vi "Add Item to Tree.vi"(7 "Tree ref":refnum<vi>, 8 "error in (no error)":errorcluster, 9 "TreeItems (to add)":T1[](array[typedef]), 10 "Insertion index":i32, 11 "TreeItems (current)":T1[](array[typedef])) -> (0 "error out":errorcluster, 3 "TreeItems (added)":T1[](array[typedef]))   [LabVIEW 2020, in "BetterDragAndDrop.lvlib" / "BetterTreeHandle.lvclass"]
uses:
  BetterTreeHandle/BetterTreeHandle.lvclass
  TreeItem.ctl
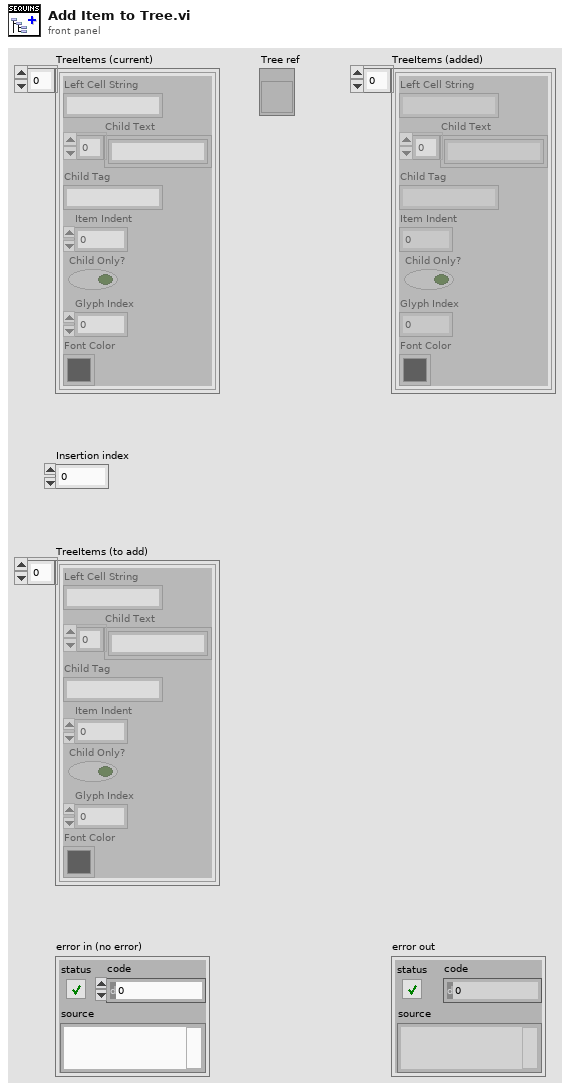
[diagram p1: front panel]
types:
  T1 = typedef "BetterDragAndDrop.lvlib/BetterTreeHandle.lvclass/TreeItem.ctl" = cluster{"Left Cell String":string, "Child Text":string[], "Child Tag":string, "Item Indent":i32, "Child Only?":bool, "Glyph Index":i32, "Font Color":u32}
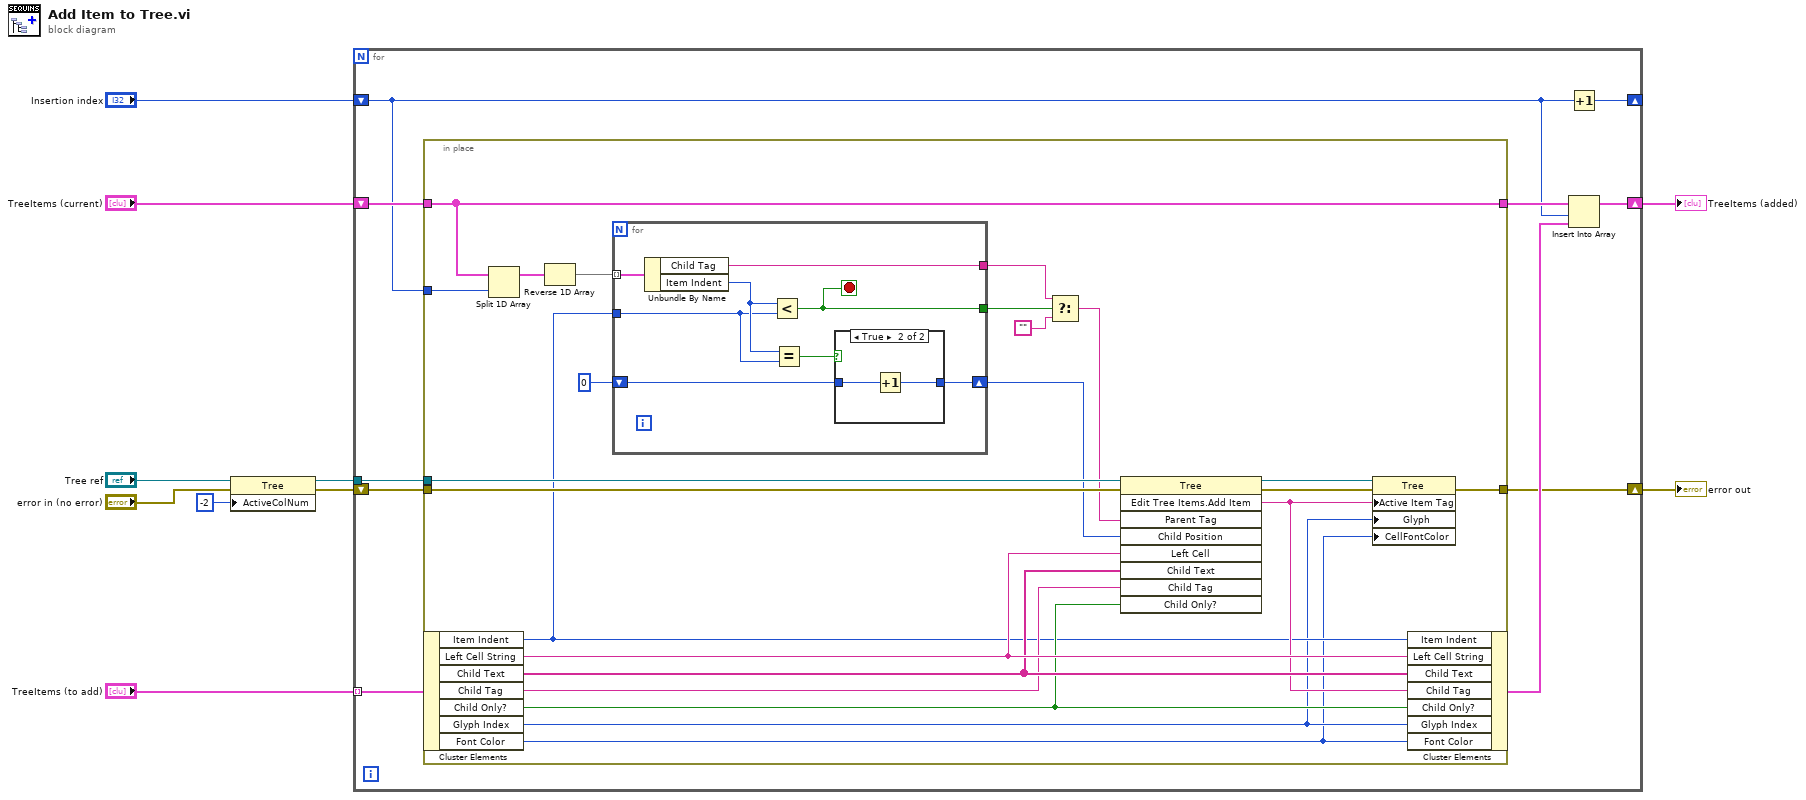
[diagram p0: block diagram]
diagram:
  n1 = property class="Tree"(reference="Tree ref", error in="error in (no error)", "ActiveColNum"=-2 ("Active Cell:Active Column Number")) -> (reference out=w2:refnum<vi>, error out=w1:errorcluster)
  n2 = for {
    tunnel: w2 -> [w20]
    shift-right: [w18] -> w6
    shift-left: "TreeItems (current)" -> [w19]
    tunnel: "TreeItems (to add)" -> [w17] mode=indexing
    shift-right: [w13] -> w7
    shift-left: w1 -> [w14]
    shift-right: [w11] -> _
    shift-left: "Insertion index" -> [w12]
    n3 = in-place {
      in-place-border: w12 -> [w43]
      in-place-border: w20 -> [w40]
      in-place-border: w19 -> [w35]
      in-place-border: [w35] -> w16
      in-place-border: w14 -> [w34]
      in-place-border: [w29] -> w13
      n4 = in-place-cluster #1(w17) -> ("Item Indent"=w31:i32, "Left Cell String"=w39:string, "Child Text"=w38:string[], "Child Tag"=w37:string, "Child Only?"=w36:bool, "Glyph Index"=w28:i32, "Font Color"=w21:u32)
      n5 = Split 1D Array(array=w35, index=w43) -> (first subarray=w42:T1[])  [unwired: 1 out]
      n6 = Reverse 1D Array(array=w42) -> (reversed array=w41:T1[])
      n7 = for {
        tunnel: w41 -> [w51] mode=indexing
        tunnel: w31 -> [w47]
        tunnel: [w50] -> w24
        tunnel: [w49] -> w25
        shift-right: [w44] -> w26
        shift-left: 0 ("Item Indent") -> [w45]
        stop <- w49 stop-if-true
        n8 = Unbundle By Name(w51) -> ("Child Tag"=w50:string, "Item Indent"=w48:i32)
        n9 = Less?(x=w48, y=w47) -> (x < y?=w49:bool)
        n10 = Equal?(x=w48, y=w47) -> (x = y?=w46:bool)
        n11 = case shown="True" w46 {
          tunnel: w45 -> [w52 w54]
          tunnel: [w52 w53] -> w44
          frame False {
          }
          frame True {
            n12 = Increment(x=w54) -> (x+1=w53:i32)
          }
        }
      }
      n13 = Select(t=w24, s=w25, f="") -> (s? t:f=w22:string)
      n14 = invoke class="Tree" method="Edit Tree Items.Add Item"(reference=w40, error in=w34, "Parent Tag"=w22, "Child Position"=w26, "Left Cell"=w39, "Child Text"=w38, "Child Tag"=w37, "Child Only?"=w36) -> (reference out=w33:refnum<vi>, error out=w30:errorcluster, "Edit Tree Items:Add Item"=w32:string)  [unwired: 1 in, 6 out]
      n15 = property class="Tree"(reference=w33, error in=w30, "Active Item Tag"=w32, "Glyph"=w28, "CellFontColor"=w21) -> (error out=w29:errorcluster)  [unwired: 1 out]
      n16 = in-place-cluster #1("Item Indent"=w31, "Left Cell String"=w39, "Child Text"=w38, "Child Tag"=w32, "Child Only?"=w36, "Glyph Index"=w28, "Font Color"=w21) -> (w15:T1)
    }
    n17 = Increment(x=w12) -> (x+1=w11:i32)
    n18 = Insert Into Array(array=w16, index=w12, new element=w15) -> (w18:T1[])
  }
  "error out" <- w7
  "TreeItems (added)" <- w6
